vi "test_main.vi"(8 "error in (no error)":errorcluster) -> (0 "error out":errorcluster)   [LabVIEW 2023]
uses:
  <vilib>/addons/_JKI Toolkits/Caraya/classes/Test/Test.lvclass
panel:
  # "Connector Pane"
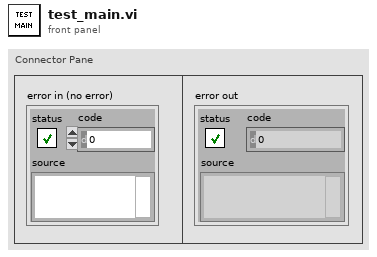
[diagram p1: front panel]
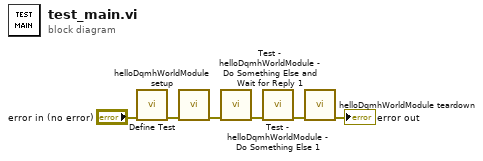
[diagram p0: block diagram]
diagram:
  n1 = call <vilib>:"Define Test.vi"("error in (no error)"="error in (no error)") -> ("error out"=w3:errorcluster)  [unwired: 9 in, 1 out]
  n2 = call "helloDqmhWorldModule setup.vi"("error in (no error)"=w3) -> ("error out"=w6:errorcluster)  [unwired: 10 in]
  n3 = call "Test - helloDqmhWorldModule - Do Something Else and Wait for Reply 1.vi"("error in"=w6) -> ("error out"=w5:errorcluster)  [unwired: 10 in]
  n4 = call "Test - helloDqmhWorldModule - Do Something Else 1.vi"("error in"=w5) -> ("error out"=w4:errorcluster)  [unwired: 10 in]
  n5 = call "helloDqmhWorldModule teardown.vi"("error in"=w4) -> ("error out"=→"error out":errorcluster)  [unwired: 10 in]
